vi "Condition Type.vi"(11 "SeqRunning Condition Config in":refnum<class "SeqRunning Condition Config.lvclass">) -> (2 "Condition Type":string)   [LabVIEW 2020, in "VolatusSeqConfig.lvlib" / "SeqRunning Condition Config.lvclass"]
uses:
  SeqRunning Condition Config.lvclass
  SeqRunning Condition Config.lvclass/SeqRunning Condition Config.ctl
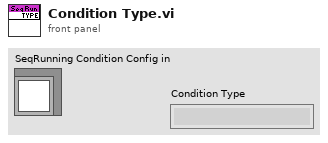
[diagram p1: front panel]
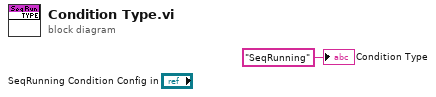
[diagram p0: block diagram]
diagram:
  "Condition Type" <- "SeqRunning" ("Condition Type")
